vi "Set VISA Resource Name.vi"(10 "VISA resource name":refnum<visa-resource-name>, 11 "GE Reflective Memory in":refnum<class "GE Reflective Memory Transceiver.lvclass">) -> (3 "GE Reflective Memory out":refnum<class "GE Reflective Memory Transceiver.lvclass">)   [LabVIEW 2020, in "GE Reflective Memory.lvlib" / "GE Reflective Memory Transceiver.lvclass"]
uses:
  GE Reflective Memory Transceiver.lvclass
  GE Reflective Memory Transceiver.lvclass/GE Reflective Memory Transceiver.ctl
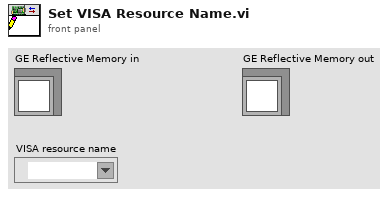
[diagram p1: front panel]
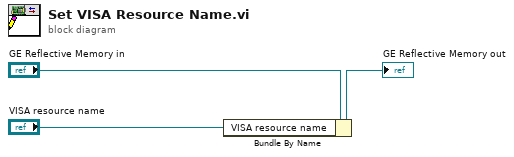
[diagram p0: block diagram]
diagram:
  n1 = Bundle By Name(cluster="GE Reflective Memory in", "VISA resource name"="VISA resource name") -> (→"GE Reflective Memory out":refnum<class "GE Reflective Memory Transceiver.lvclass">)
